vi "VISA_IDN.vi"(0 "Session In":refnum<visa-resource-name>="TCPIP0::10.0.1.24::inst0::INSTR", 5 "error in":errorcluster {"code" format="%.0x"}, 6 "INST(name)":string) -> (13 "concatenated string":string, 14 "Session Out":refnum<visa-resource-name>, 15 "Mfr":string, 16 "Model":string, 17 "Ver":string, 18 "SN":string, 19 "error out":errorcluster {"code" format="%.0x"})   [LabVIEW 2018]
panel:
  out "Address":string
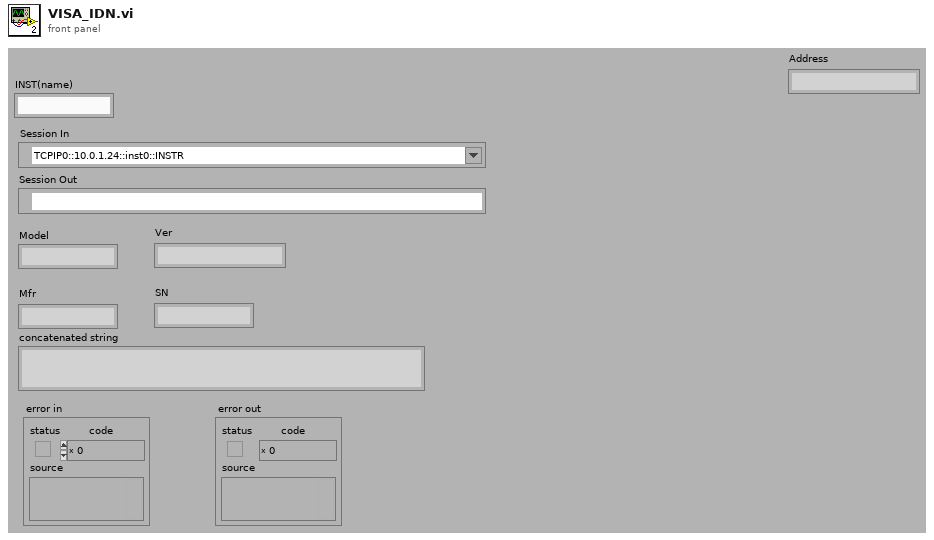
[diagram p1: front panel]
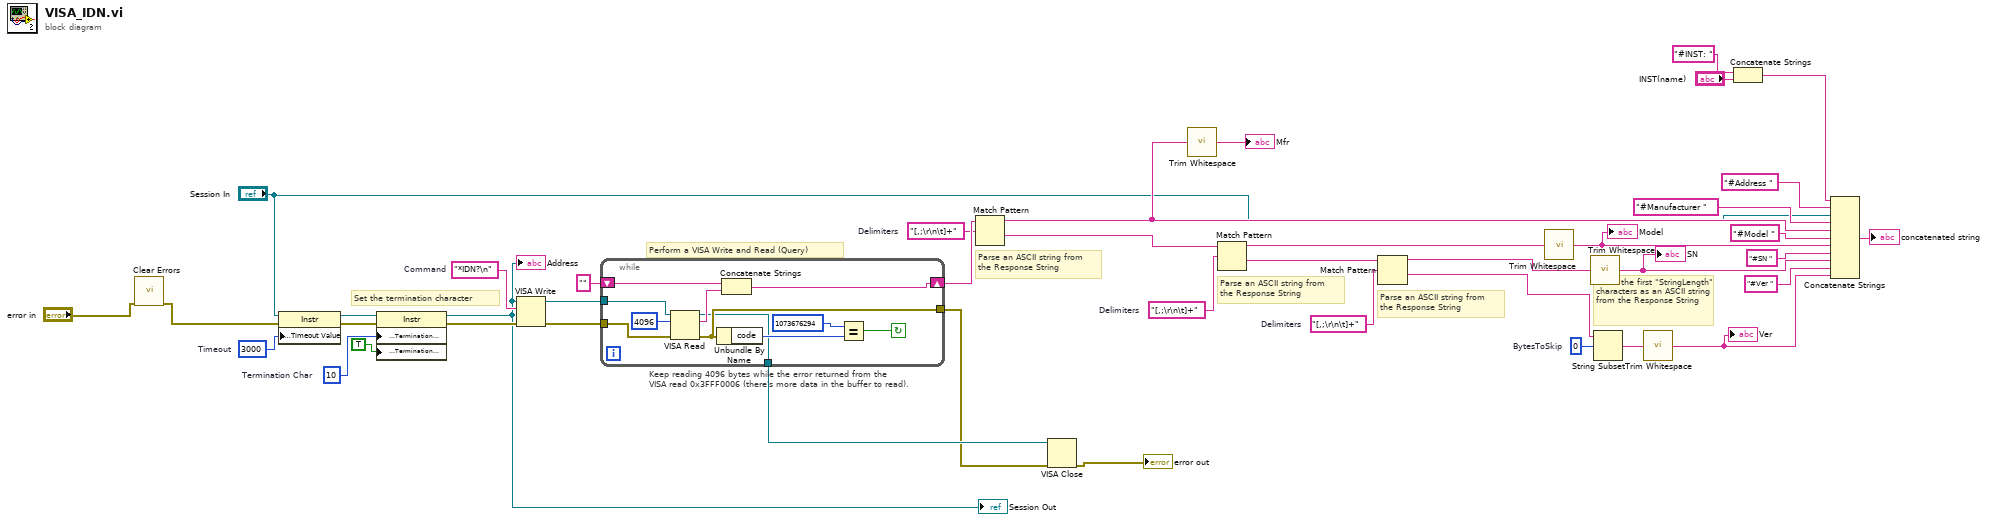
[diagram p0: block diagram]
diagram:
  w25 = 0  # BytesToSkip
  w26 = "[,;\r\n\t]+"  # Delimiters
  w28 = "[,;\r\n\t]+"  # Delimiters
  w30 = "[,;\r\n\t]+"  # Delimiters
  w32 = "*IDN?\n"  # Command
  w38 = u8 10  # Termination Char
  w42 = u32 3000  # Timeout
  # "Parse the first \"StringLength\" characters as an ASCII string from the Response String"
  # "Parse an ASCII string from the Response String"
  # "Parse an ASCII string from the Response String"
  # "Parse an ASCII string from the Response String"
  # "Perform a VISA Write and Read (Query)"
  # "Keep reading 4096 bytes while the error returned from the\nVISA read 0x3FFF0006 (there's more data in the buffer to read)."
  # "Set the termination character"
  n1 = call <vilib>:"Clear Errors.vi"("error in (no error)"="error in") -> ("error out"=w1:errorcluster)  [unwired: 5 in, 1 out]
  n2 = property class="Instr"(reference="Session In", error in=w1, "General Settings:Timeout Value"=w42) -> (reference out=w41:refnum<visa-resource-name>, error out=w40:errorcluster)
  n3 = property class="Instr"(reference=w41, error in=w40, "Message Based Settings:Termination Character"=w38, "Message Based Settings:Termination Character Enable"=TRUE ("enable")) -> (reference out=w13:refnum<visa-resource-name>, error out=w39:errorcluster)
  "Session Out" <- w13
  "Address" <- w13
  n4 = VISA Write(VISA resource name=w13, write buffer=w32, error in (no error)=w39) -> (VISA resource name out=w36:refnum<visa-resource-name>, error out=w34:errorcluster)  [unwired: 1 out]
  n5 = while {
    tunnel: w36 -> [w50]
    shift-right: [w44] -> w35
    shift-left: "" -> [w49]
    tunnel: w34 -> [w47]
    tunnel: [w46] -> w11
    tunnel: [w43] -> w12
    stop <- w45 continue-if-true
    n6 = VISA Read(VISA resource name=w50, byte count=u32 4096 ("byte count (0)"), error in (no error)=w47) -> (VISA resource name out=w43:refnum<visa-resource-name>, read buffer=w48:string, error out=w46:errorcluster)  [unwired: 1 out]
    n7 = Unbundle By Name(w46) -> ("code"=w52:i32)
    n8 = Concatenate Strings(w49, w48) -> (w44:string)
    n9 = Equal?(x=1073676294, y=w52) -> (x = y?=w45:bool)
  }
  n10 = Match Pattern(string=w35, regular expression=w30) -> (before substring=w20:string, after substring=w31:string)  [unwired: 1 in, 2 out]
  n11 = VISA Close(VISA resource name=w12, error in (no error)=w11) -> (error out=→"error out":errorcluster)
  n12 = call <vilib>:"Trim Whitespace.vi"("string"=w20) -> ("trimmed string"=→"Mfr":string)  [unwired: 1 in]
  n13 = Match Pattern(string=w31, regular expression=w28) -> (before substring=w24:string, after substring=w29:string)  [unwired: 1 in, 2 out]
  n14 = Match Pattern(string=w29, regular expression=w26) -> (before substring=w17:string, after substring=w27:string)  [unwired: 1 in, 2 out]
  n15 = call <vilib>:"Trim Whitespace.vi"("string"=w24) -> ("trimmed string"=w6:string)  [unwired: 1 in]
  "Model" <- w6
  n16 = call <vilib>:"Trim Whitespace.vi"("string"=w17) -> ("trimmed string"=w5:string)  [unwired: 1 in]
  "SN" <- w5
  n17 = String Subset(string=w27, offset (0)=w25) -> (substring=w15:string)  [unwired: 1 in]
  n18 = call <vilib>:"Trim Whitespace.vi"("string"=w15) -> ("trimmed string"=w4:string)  [unwired: 1 in]
  "Ver" <- w4
  n19 = Concatenate Strings("#INST: " ("string"), "INST(name)") -> (w9:string)
  n20 = Concatenate Strings(w9, "#Address " ("string"), "Session In", "#Manufacturer ", w20, "#Model ", w6, "#SN " ("string"), w5, "#Ver " ("string"), w4) -> (→"concatenated string":string)
